vi "Verify_Single.vi"(8 "error in":errorcluster, 10 "Switch ID":i32, 11 "Switch Functin":enum16{"Open Switch", "Closed Switch"}(ring)) -> (0 "Error out":errorcluster, 3 "Verfied":bool)   [LabVIEW 2012]
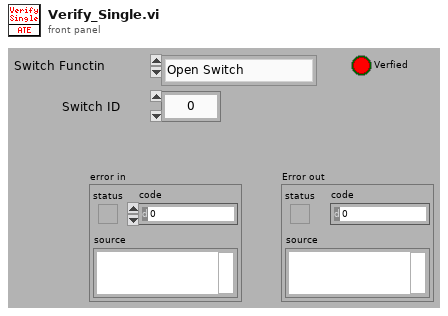
[diagram p1: front panel]
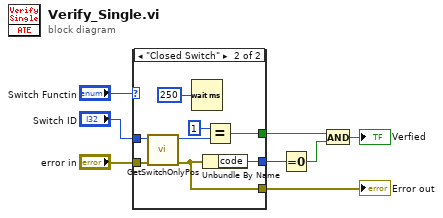
[diagram p0: block diagram]
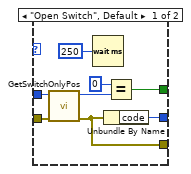
[diagram p2: hidden frame]
diagram:
  n1 = case shown="\"Closed Switch\"" "Switch Functin" {
    tunnel: [w13 w22] -> w3
    tunnel: "error in" -> [w14 w21]
    tunnel: [w12 w20] -> w5
    tunnel: "Switch ID" -> [w10 w19]
    tunnel: [w9 w17] -> w1
    frame "Open Switch", Default {
      n2 = call "GetSwitchOnlyPos.vi"("error in (no error)"=w14, "Circuit ID"=w10) -> ("Error out"=w9:errorcluster, "Position (0=open, 1=closed)"=w15:i32)  [unwired: 4 in]
      n3 = Wait (ms)(milliseconds to wait=u32 250) -> ()  [unwired: 1 out]
      n4 = Unbundle By Name(w9) -> ("code"=w12:i32)
      n5 = Equal?(x=0 ("Position (0=open, 1=closed)"), y=w15) -> (x = y?=w13:bool)
    }
    frame "Closed Switch" {
      n6 = call "GetSwitchOnlyPos.vi"("error in (no error)"=w21, "Circuit ID"=w19) -> ("Error out"=w17:errorcluster, "Position (0=open, 1=closed)"=w24:i32)  [unwired: 4 in]
      n7 = Wait (ms)(milliseconds to wait=u32 250) -> ()  [unwired: 1 out]
      n8 = Unbundle By Name(w17) -> ("code"=w20:i32)
      n9 = Equal?(x=1 ("Position (0=open, 1=closed)"), y=w24) -> (x = y?=w22:bool)
    }
  }
  "Error out" <- w1
  n10 = Equal To 0?(x=w5) -> (x = 0?=w8:bool)
  n11 = And(x=w3, y=w8) -> (x .and. y?=→"Verfied":bool)
